vi "PH_Periodic_Sequencer.ProcPeriodic.vi"(0 "i ref in":refnum<vi>, 3 "ms timeout (100)":i32=100, 5 "error in (no error)":errorcluster) -> (14 "i ref out":refnum<vi>, 17 "timed out":bool, 19 "error out":errorcluster)   [LabVIEW 2014, in "PH_Periodic_Sequencer.lvlib"]
doc: "This method serves to periodically do things like reading values from the HW. Methods that should be executed periodically should be called from THIS methode. Add code here."
uses:
  PH_Periodic_Sequencer.lvlib
  PH_StatusHandler/PH_StatusHandler.Status.ctl
  PH_Sequencer/PH_Sequencer.lvlib
  PH_StatusHandler/PH_StatusHandler.lvlib
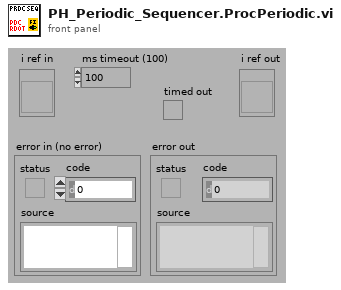
[diagram p1: front panel]
types:
  T1 = typedef "PH_Periodic_Sequencer.lvlib/PH_Periodic_Sequencer.i attribute.ctl" = cluster{"GUI Refs":cluster{"Main Off":refnum<vi>, "Start":refnum<vi>, "Ready":refnum<vi>, "Sequencer SM State":refnum<vi>, "Interval [sec]":refnum<vi>, "Wanted Shots":refnum<vi>, "Delivered Shots":refnum<vi>}, "PU Info":cluster{"Instancename":string, "State":T2, "linked":bool}[], "Sequencer":cluster{"Instancename":string, "linked?":bool, "R2S?":bool, "SM State":string}, "Run?":bool, "Interval [sec]":dbl, "PU State Refs":refnum<vi>[], "Wanted Shots":i32, "Delivered Shots":i32}
  T2 = typedef "PH_StatusHandler.lvlib/PH_StatusHandler.Status.ctl" = i16
  T3 = cluster{"Instancename":string, "State":T2, "linked":bool}[]
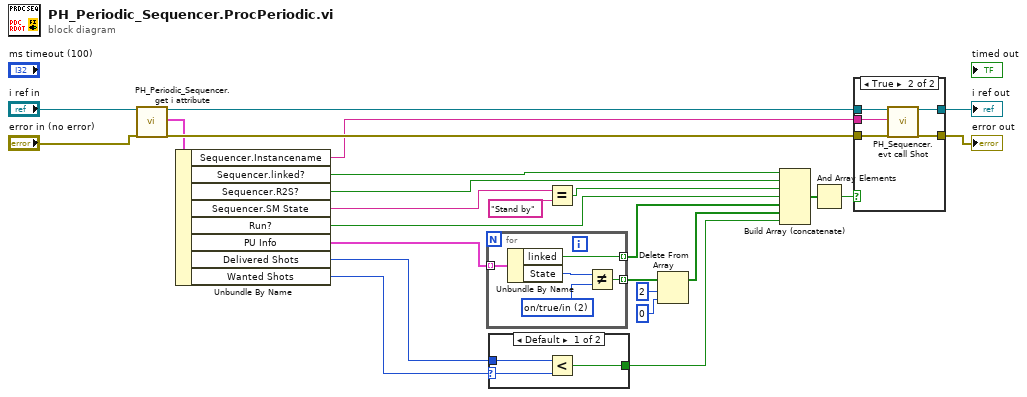
[diagram p0: block diagram]
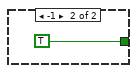
[diagram p2: hidden frame]
diagram:
  n1 = call "PH_Periodic_Sequencer.get i attribute.vi"("i ref in"="i ref in", "error in (no error)"="error in (no error)") -> ("i ref out"=w22:refnum<vi>, "i attribute"=w19:T1, "error out"=w20:errorcluster)  [unwired: 15 in]
  n2 = Unbundle By Name(w19) -> ("Sequencer.Instancename"=w18:string, "Sequencer.linked?"=w17:bool, "Sequencer.R2S?"=w16:bool, "Sequencer.SM State"=w13:string, "Run?"=w12:bool, "PU Info"=w11:T3, "Delivered Shots"=w1:i32, "Wanted Shots"=w2:i32)
  n3 = for {
    tunnel: w11 -> [w30] mode=indexing
    tunnel: [w29] -> w10 mode=indexing
    tunnel: [w26] -> w9 mode=indexing
    w27 = T2 2 items=["no info", "off/false/out", "on/true/in", "Failure", "Alarm", "Status 1", "Status 2", "Status 3"] ("y")
    n4 = Unbundle By Name(w30) -> ("linked"=w29:bool, "State"=w28:T2)
    n5 = Not Equal?(x=w28, y=w27) -> (x != y?=w26:bool)
  }
  n6 = case shown="Default" w2 {
    selector: w2 -> [w32 _]
    tunnel: [w31 TRUE] -> w3
    tunnel: w1 -> [w33 _]
    frame Default {
      n7 = Less?(x=w33, y=w32) -> (x < y?=w31:bool)
    }
    frame -1 {
    }
  }
  n8 = Equal?(x=w13, y="Stand by") -> (x = y?=w14:bool)
  n9 = Delete From Array(array=w9, length=2, index=0) -> (array with subset deleted=w6:bool[])  [unwired: 1 out]
  n10 = Build Array (concatenate)(w17, w16, w14, w12, w10, w6, w3) -> (w5:bool[])
  n11 = And Array Elements(Boolean array=w5) -> (logical AND=w4:bool)
  n12 = case shown="True" w4 {
    tunnel: [w35 w41] -> w25
    tunnel: [w36 w40] -> w24
    tunnel: w22 -> [w36 w39]
    tunnel: w20 -> [w35 w38]
    tunnel: w18 -> [_ w37]
    frame False {
    }
    frame True {
      n13 = call "PH_Sequencer.evt call Shot.vi"("i ref in"=w39, "Sequencer Instance"=w37, "error in (no error)"=w38) -> ("i ref out"=w40:refnum<vi>, "error out"=w41:errorcluster)  [unwired: 15 in]
    }
  }
  "error out" <- w25
  "i ref out" <- w24
